vi "launch background process.vi"(7 "execution period (ms)":i32, 8 "error in":errorcluster, 9 "data allocations":T3, 10 "execution settings":T1, 11 "module runtime":refnum<class "TBM module execution interface.lvclass">) -> (0 "error out":errorcluster, 3 "async data":T2)   [LabVIEW 2013, in "Standard Engine Runtime.lvclass"]
uses:
  Standard Engine Runtime.lvclass
  <vilib>/NI/Tag Bus Module Framework/channel/data tables.ctl
  <vilib>/NI/Tag Bus/dictionary/data dictionary.lvclass
  <vilib>/NI/Tag Bus/dictionary table pair.ctl
  <vilib>/NI/Tag Bus/table/data table.ctl
  asynchronous process data.ctl
  async command notification.ctl
  <vilib>/NI/Tag Bus Module Framework/runtime/execution settings.ctl
  async error info.ctl
  <vilib>/NI/Tag Bus Module Framework/runtime/error classification.ctl
  <vilib>/NI/Tag Bus Module Framework/runtime/TBM module execution interface.lvclass
  asynchronous background process.vi
  <vilib>/NI/Tag Bus/table/data table.lvlib
  <vilib>/NI/Tag Bus/tag bus.lvlib
  <vilib>/NI/Tag Bus Module Framework/channel/TBM channel.lvclass
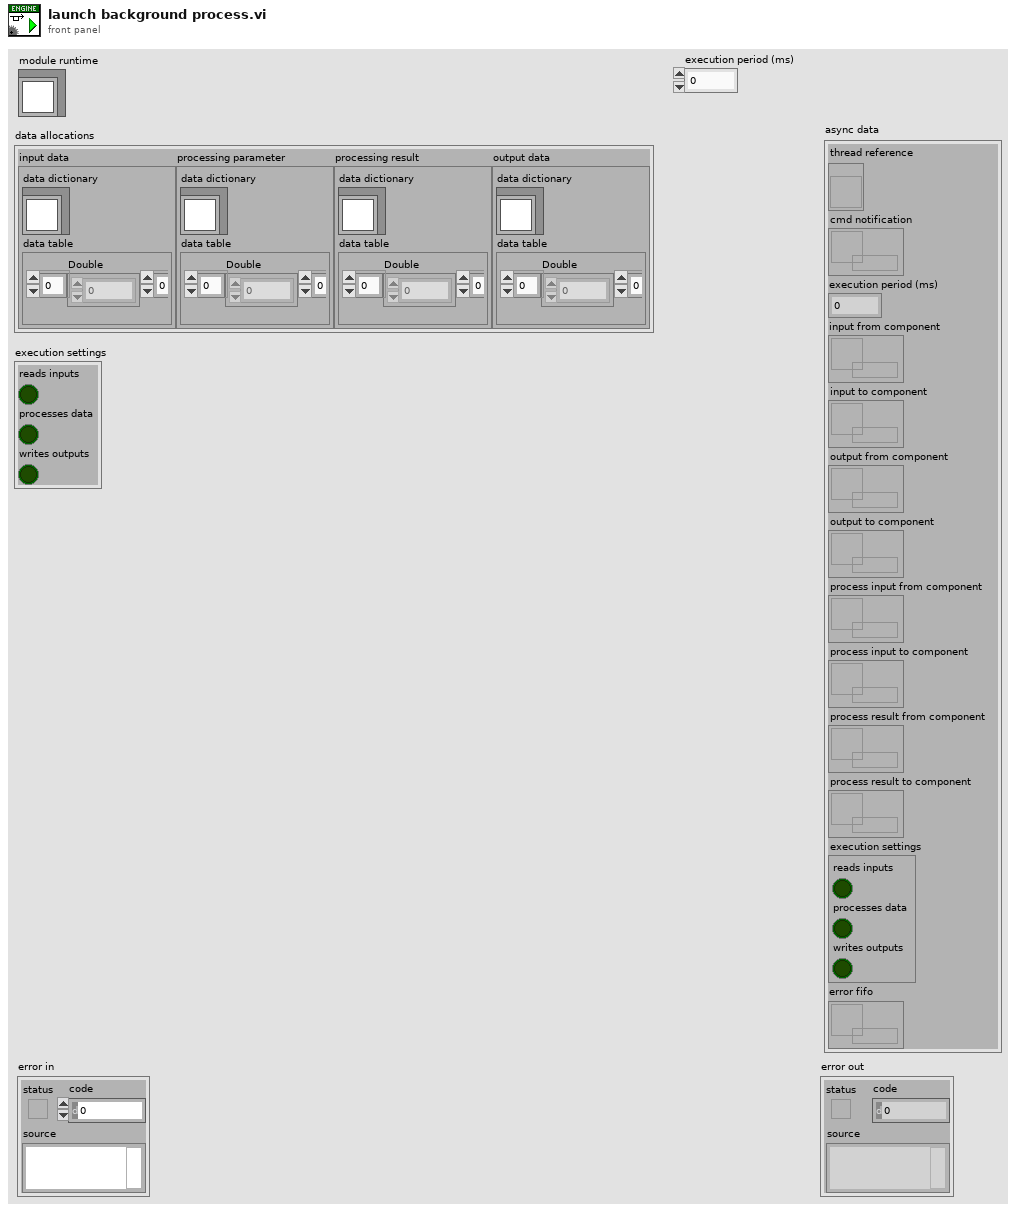
[diagram p1: front panel]
types:
  T1 = typedef "TBM module execution interface.lvclass/execution settings.ctl" = cluster{"reads inputs":bool, "processes data":bool, "writes outputs":bool}
  T2 = typedef "Standard Engine Runtime.lvclass/asynchronous process data.ctl" = cluster{"thread reference":refnum<vi>, "cmd notification":refnum<k33>, "execution period (ms)":i32, "input from component":refnum<queue>, "input to component":refnum<queue>, "output from component":refnum<queue>, "output to component":refnum<queue>, "process input from component":refnum<queue>, "process input to component":refnum<queue>, "process result from component":refnum<queue>, "process result to component":refnum<queue>, "execution settings":T1, "error fifo":refnum<k33>}
  T3 = typedef "TBM channel.lvclass/data tables.ctl" = cluster{"input data":T4, "processing parameter":T4, "processing result":T4, "output data":T4}
  T4 = typedef "tag bus.lvlib/dictionary table pair.ctl" = cluster{"data dictionary":refnum<class "data dictionary.lvclass">, "data table":T5}
  T5 = typedef "tag bus.lvlib/data table.lvlib/data table.ctl" = cluster{"Double":dbl[], "Single":sgl[], "I64":i64[], "I32":i32[], "I16":i16[], "I8":i8[], "U64":u64[], "U32":u32[], "U16":u16[], "U8":u8[], "Boolean":bool[], "String":string[], "Array of Double":cluster{"DBL Array":dbl[]}[], "Array of Single":cluster{"SGL Array":sgl[]}[], "Array of I64":cluster{"I64 Array":i64[]}[], "Array of I32":cluster{"I32 Array":i32[]}[], "Array of I16":cluster{"I16 Array":i16[]}[], "Array of I8":cluster{"I8 Array":i8[]}[], "Array of U64":cluster{"U64 Array":u64[]}[], "Array of U32":cluster{"U32 Array":u32[]}[], "Array of U16":cluster{"U16 Array":u16[]}[], "Array of U8":cluster{"U8 Array":u8[]}[], "Array of Boolean":cluster{"Boolean Array":bool[]}[], "Array of String":cluster{"String Array":string[]}[]}
  T6 = typedef "Standard Engine Runtime.lvclass/async error info.ctl" = cluster{"error code":i32, "error classification":T7}
  T7 = typedef "TBM module execution interface.lvclass/error classification.ctl" = enum16{"unknown", "none", "trivial", "recoverable", "critical"}
  T8 = typedef "Standard Engine Runtime.lvclass/async command notification.ctl" = enum16{"stop", "safe state", "recover", "clear error"}
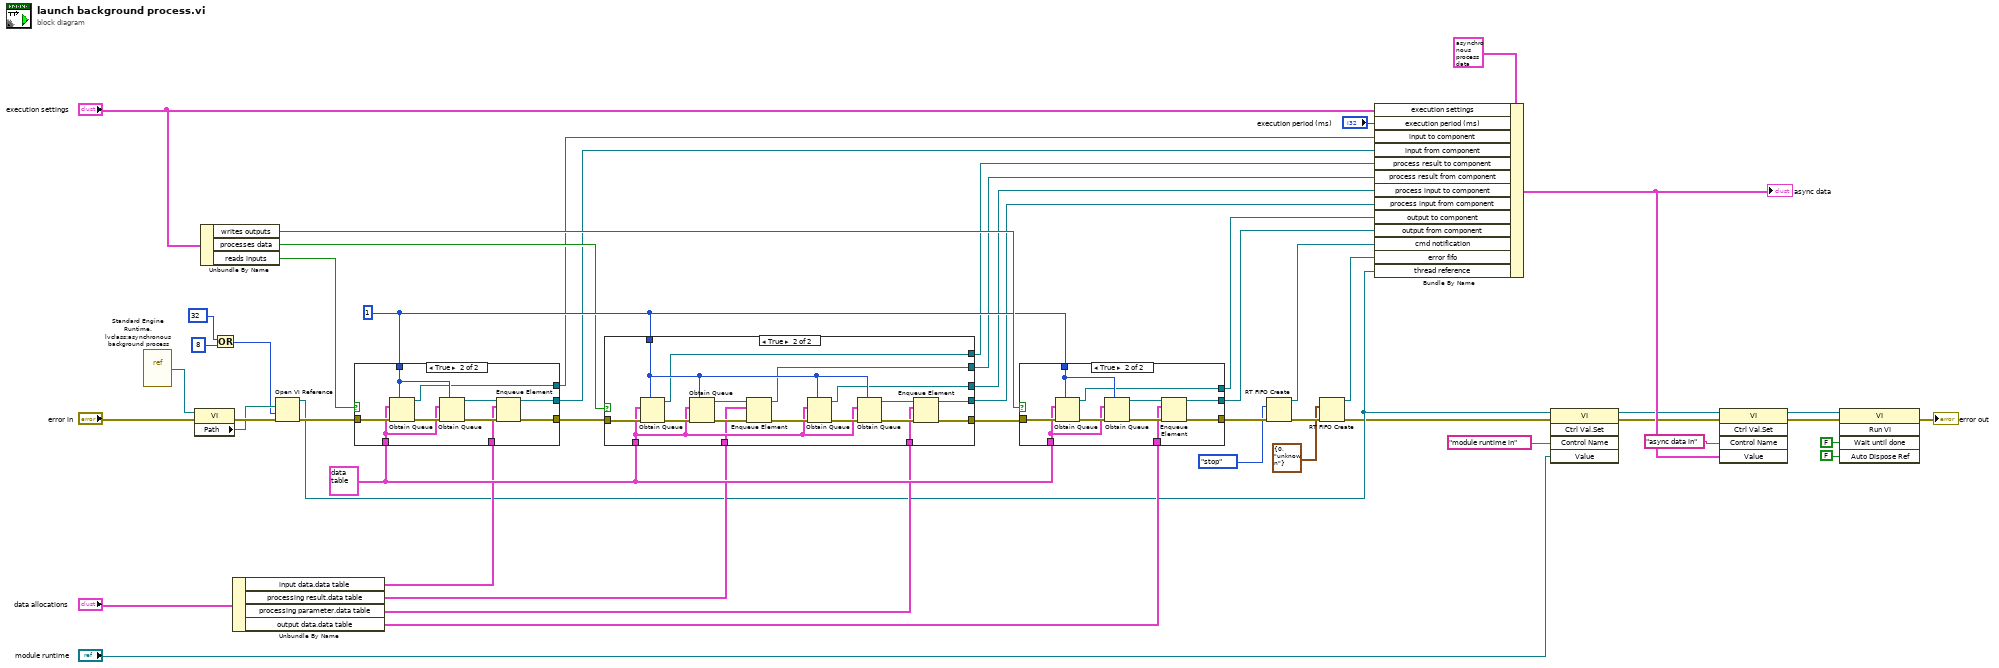
[diagram p0: block diagram]
diagram:
  w25 = 1 ("max queue size (-1, unlimited)")
  w26 = T5 {"Double"=[], "Single"=[], "I64"=[], "I32"=[], "I16"=[], "I8"=[], "U64"=[], "U32"=[], "U16"=[], "U8"=[], "Boolean"=[], "String"=[], "Array of Double"=[], "Array of Single"=[], "Array of I64"=[], "Array of I32"=[], "Array of I16"=[], "Array of I8"=[], "Array of U64"=[], "Array of U32"=[], "Array of U16"=[], "Array of U8"=[], "Array of Boolean"=[], "Array of String"=[]} ("input data")
  n1 = vi-ref "Standard Engine Runtime.lvclass:asynchronous background process.vi"() -> (w48:refnum<vi>)
  n2 = property class="VI"(reference=w48, error in="error in") -> (error out=w49:errorcluster, "Path"=w47:path)  [unwired: 1 out]
  n3 = Unbundle By Name("execution settings") -> ("writes outputs"=w29:bool, "processes data"=w24:bool, "reads inputs"=w31:bool)
  n4 = Or(x=32 ("options"), y=8 ("options")) -> (x .or. y?=w36:i32)
  n5 = Unbundle By Name("data allocations") -> ("input data.data table"=w15:T5, "processing result.data table"=w12:T5, "processing parameter.data table"=w13:T5, "output data.data table"=w14:T5)
  n6 = Open VI Reference(vi path=w47, options=w36, error in (no error)=w49) -> (vi reference=w10:refnum<vi>, error out=w32:errorcluster)  [unwired: 3 in]
  n7 = case shown="True" w31 {
    tunnel: w32 -> [w51 w58]
    tunnel: [w51 w57] -> w28
    tunnel: w26 -> [_ w56]
    tunnel: w25 -> [_ w55]
    tunnel: [_ w54] -> w22
    tunnel: [_ w53] -> w23
    tunnel: w15 -> [_ w52]
    frame False {
    }
    frame True {
      n8 = Obtain Queue(max queue size (-1, unlimited)=w55, element data type=w56, error in (no error)=w58) -> (queue out=w53:refnum<queue>, error out=w61:errorcluster)  [unwired: 2 in, 1 out]
      n9 = Obtain Queue(max queue size (-1, unlimited)=w55, element data type=w56, error in (no error)=w61) -> (queue out=w59:refnum<queue>, error out=w60:errorcluster)  [unwired: 2 in, 1 out]
      n10 = Enqueue Element(queue=w59, element=w52, error in (no error)=w60) -> (queue out=w54:refnum<queue>, error out=w57:errorcluster)  [unwired: 1 in, 1 out]
    }
  }
  n11 = case shown="True" w24 {
    tunnel: w28 -> [w62 w76]
    tunnel: [w62 w71] -> w27
    tunnel: w26 -> [_ w69]
    tunnel: w25 -> [_ w70]
    tunnel: [_ w68] -> w21
    tunnel: [_ w67] -> w20
    tunnel: [_ w66] -> w19
    tunnel: [_ w65] -> w18
    tunnel: w13 -> [_ w64]
    tunnel: w12 -> [_ w63]
    frame False {
    }
    frame True {
      n12 = Obtain Queue(max queue size (-1, unlimited)=w70, element data type=w69, error in (no error)=w76) -> (queue out=w65:refnum<queue>, error out=w79:errorcluster)  [unwired: 2 in, 1 out]
      n13 = Obtain Queue(max queue size (-1, unlimited)=w70, element data type=w69, error in (no error)=w79) -> (queue out=w77:refnum<queue>, error out=w78:errorcluster)  [unwired: 2 in, 1 out]
      n14 = Enqueue Element(queue=w77, element=w63, error in (no error)=w78) -> (queue out=w66:refnum<queue>, error out=w72:errorcluster)  [unwired: 1 in, 1 out]
      n15 = Obtain Queue(max queue size (-1, unlimited)=w70, element data type=w69, error in (no error)=w72) -> (queue out=w67:refnum<queue>, error out=w73:errorcluster)  [unwired: 2 in, 1 out]
      n16 = Obtain Queue(max queue size (-1, unlimited)=w70, element data type=w69, error in (no error)=w73) -> (queue out=w75:refnum<queue>, error out=w74:errorcluster)  [unwired: 2 in, 1 out]
      n17 = Enqueue Element(queue=w75, element=w64, error in (no error)=w74) -> (queue out=w68:refnum<queue>, error out=w71:errorcluster)  [unwired: 1 in, 1 out]
    }
  }
  n18 = case shown="True" w29 {
    tunnel: w27 -> [w80 w87]
    tunnel: [w80 w86] -> w30
    tunnel: w26 -> [_ w85]
    tunnel: w25 -> [_ w84]
    tunnel: [_ w83] -> w17
    tunnel: [_ w82] -> w16
    tunnel: w14 -> [_ w81]
    frame False {
    }
    frame True {
      n19 = Obtain Queue(max queue size (-1, unlimited)=w84, element data type=w85, error in (no error)=w87) -> (queue out=w82:refnum<queue>, error out=w90:errorcluster)  [unwired: 2 in, 1 out]
      n20 = Obtain Queue(max queue size (-1, unlimited)=w84, element data type=w85, error in (no error)=w90) -> (queue out=w88:refnum<queue>, error out=w89:errorcluster)  [unwired: 2 in, 1 out]
      n21 = Enqueue Element(queue=w88, element=w81, error in (no error)=w89) -> (queue out=w83:refnum<queue>, error out=w86:errorcluster)  [unwired: 1 in, 1 out]
    }
  }
  n22 = RT FIFO Create(1:async_command_notification."stop" ("async command"), 3:w30) -> (8:w1:refnum<k33>, 11:w5:errorcluster)  [unwired: 6 in, 1 out]
  n23 = RT FIFO Create(1:T6 {"error code"=0, "error classification"=enum."unknown"}, 3:w5) -> (8:w2:refnum<k33>, 11:w4:errorcluster)  [unwired: 6 in, 1 out]
  n24 = Bundle By Name(cluster=T2 {"thread reference"=refnum, "cmd notification"=refnum, "execution period (ms)"=0, "input from component"=refnum, "input to component"=refnum, "output from component"=refnum, "output to component"=refnum, "process input from component"=refnum, "process input to component"=refnum, "process result from component"=refnum, "process result to component"=refnum, "execution settings"={"reads inputs"=FALSE, "processes data"=FALSE, "writes outputs"=FALSE}, "error fifo"=refnum} ("async data"), "execution settings"="execution settings", "execution period (ms)"="execution period (ms)", "input to component"=w23, "input from component"=w22, "process result to component"=w18, "process result from component"=w19, "process input to component"=w20, "process input from component"=w21, "output to component"=w16, "output from component"=w17, "cmd notification"=w1, "error fifo"=w2, "thread reference"=w10) -> (w37:T2)
  "async data" <- w37
  n25 = invoke class="VI" method="Ctrl Val.Set"(reference=w10, error in=w4, "Control Name"="module runtime in", "Value"="module runtime") -> (reference out=w9:refnum<vi>, error out=w11:errorcluster)  [unwired: 1 in, 3 out]
  n26 = invoke class="VI" method="Ctrl Val.Set"(reference=w9, error in=w11, "Control Name"="async data in", "Value"=w37) -> (reference out=w45:refnum<vi>, error out=w44:errorcluster)  [unwired: 1 in, 3 out]
  n27 = invoke class="VI" method="Run VI"(reference=w45, error in=w44, "Wait until done"=FALSE ("Wait Until Done"), "Auto Dispose Ref"=FALSE ("Auto Dispose Reference")) -> (error out=→"error out":errorcluster)  [unwired: 1 in, 4 out]
